vi "Sections Get Data.vi"(8 "Error In":errorcluster) -> (0 "Error Out":errorcluster, 1 "TotalPrice (Footer)":dbl, 3 "Line Items":T1[](array[typedef]) {"PriceIncDiscount (£)" format="%.2g"; "Discount(£)" format="%.2g"}, 4 "DateTime (Footer)":timestamp, 5 "Location":string)   [LabVIEW 2018, in "Receipt Parsing.lvlib"]
uses:
  Receipt Parsing.lvlib
  main/ReceiptItemInfo.ctl
  Action.ctl
  Provisional Parsed Values--cluster.ctl
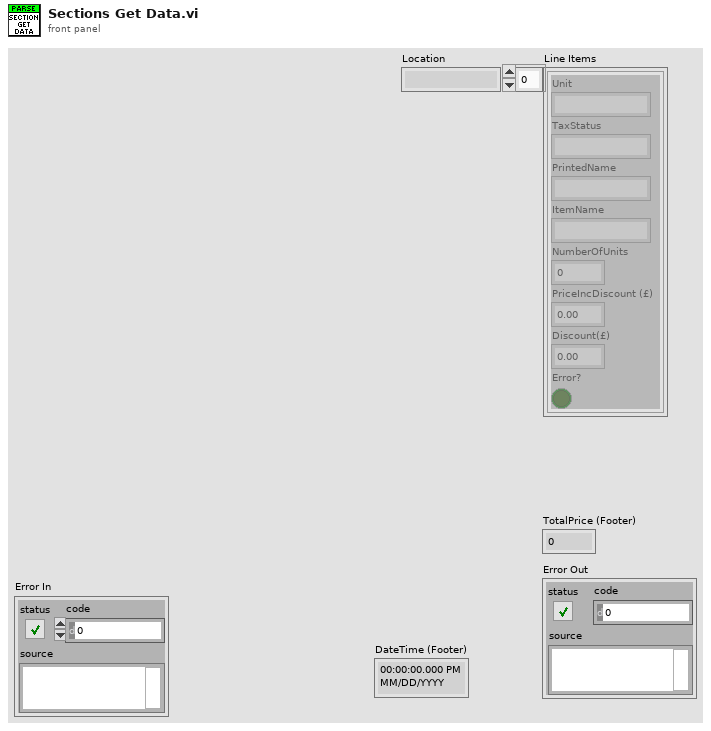
[diagram p1: front panel]
types:
  T1 = typedef "Receipt Parsing.lvlib/ReceiptItemInfo.ctl" = cluster{"Unit":string, "TaxStatus":string, "PrintedName":string, "ItemName":string, "NumberOfUnits":dbl, "PriceIncDiscount (£)":dbl, "Discount(£)":dbl, "Error?":bool}
  T2 = typedef "Receipt Parsing.lvlib/Provisional Parsed Values--cluster.ctl" = cluster{"Location":string, "Line Items ":T1[], "TotalPrice":dbl, "DateTime":timestamp}
  T3 = typedef "Receipt Parsing.lvlib/Action.ctl" = enum16{"Init", "Read Image Text", "Text Get Sections", "Sections Get Data", "Close"}
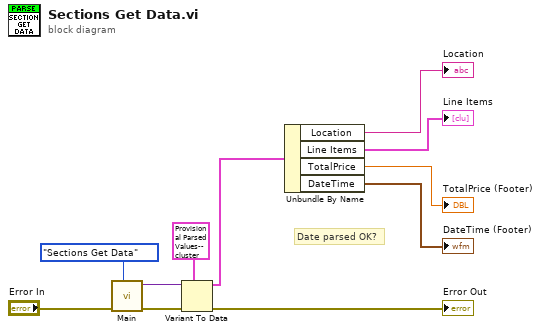
[diagram p0: block diagram]
diagram:
  # "Date parsed OK?"
  n1 = call "Main.vi"("Action"=Action."Sections Get Data", "Error In"="Error In") -> ("Error Out"=w6:errorcluster, "Data Out"=w9:variant)  [unwired: 8 in]
  n2 = Variant To Data(error in=w6, type=T2 {"Location"="", "Line Items "=[], "TotalPrice"=0.0, "DateTime"=timestamp(0 s since 1904-01-01)} ("Provisional Parsed Values"), Variant=w9) -> (data=w5:T2, error out=→"Error Out":errorcluster)
  n3 = Unbundle By Name(w5) -> ("Location"=→"Location":string, "Line Items"=→"Line Items":T1[], "TotalPrice"=→"TotalPrice (Footer)":dbl, "DateTime"=→"DateTime (Footer)":timestamp)
